vi "u16.to.bytes.vi"(11 "data.u16.in":u16[](array[numeric])=[0, 0, 0, 0, 0, 0, 0, 0]) -> ()   [LabVIEW 2020, in "fpganow.common.fpga.lvlib"]
uses:
  fpganow.common.fpga.lvlib
  u64.data.ctl
panel:
  out "data":T1 {"byte" format="%.0x"}
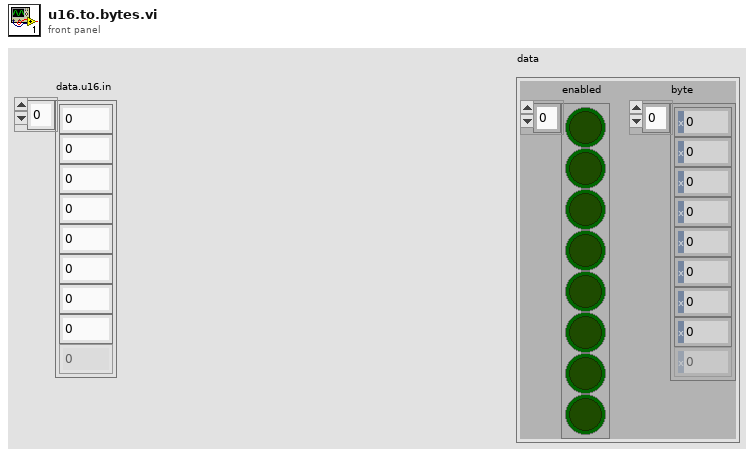
[diagram p1: front panel]
types:
  T1 = typedef "fpganow.common.fpga.lvlib/u64.data.ctl" = cluster{"enabled":bool[], "byte":u8[]}
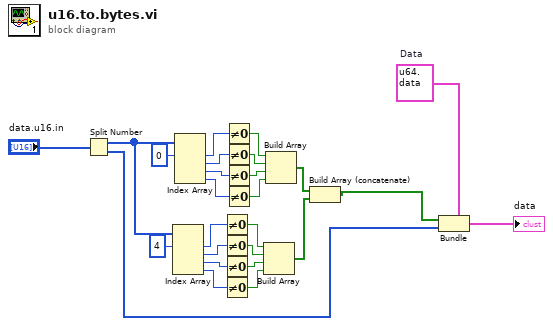
[diagram p0: block diagram]
diagram:
  w2 = T1 {"enabled"=[FALSE, FALSE, FALSE, FALSE, FALSE, FALSE, FALSE, FALSE], "byte"=[0, 0, 0, 0, 0, 0, 0, 0]}  # Data
  n1 = Split Number(x="data.u16.in") -> (hi(x)=w23:u8[], lo(x)=w3:u8[])
  n2 = Index Array(array=w23, index #1=4 ("index")) -> (element #1=w25:u8, element #2=w17:u8, element #3=w18:u8, element #4=w19:u8)  [unwired: 3 in]
  n3 = Index Array(array=w23, index #1=0 ("index")) -> (element #1=w7:u8, element #2=w8:u8, element #3=w9:u8, element #4=w10:u8)  [unwired: 3 in]
  n4 = Not Equal To 0?(x=w25) -> (x != 0?=w26:bool)
  n5 = Not Equal To 0?(x=w17) -> (x != 0?=w22:bool)
  n6 = Not Equal To 0?(x=w18) -> (x != 0?=w21:bool)
  n7 = Not Equal To 0?(x=w19) -> (x != 0?=w20:bool)
  n8 = Not Equal To 0?(x=w7) -> (x != 0?=w12:bool)
  n9 = Not Equal To 0?(x=w8) -> (x != 0?=w15:bool)
  n10 = Not Equal To 0?(x=w9) -> (x != 0?=w14:bool)
  n11 = Not Equal To 0?(x=w10) -> (x != 0?=w13:bool)
  n12 = Build Array(w26, w22, w21, w20) -> (w24:bool[])
  n13 = Build Array(w12, w15, w14, w13) -> (w11:bool[])
  n14 = Build Array (concatenate)(w11, w24) -> (w4:bool[])
  n15 = Bundle(cluster=w2, "enabled"=w4, "byte"=w3) -> (→"data":T1)
